vi "Set_Pulse_Single_Channel.vi"(0 "VISA arduino in":refnum<visa-resource-name>, 1 "chanel":u8=2 min=2 max=13 step=1, 2 "Times":dbl[](array[numeric]), 3 "error in":errorcluster, 4 "Check times?":bool) -> (5 "VISA arduino out":refnum<visa-resource-name>, 6 "error out":errorcluster)   [LabVIEW 2021]
uses:
  Delay_Global.vi
  <vilib>/Utility/error.llb/Error Cluster From Error Code.vi
  <vilib>/ErrorRing/Error Ring.xnode
panel:
  out "delay":u32
  # "Private"
  # "Public"
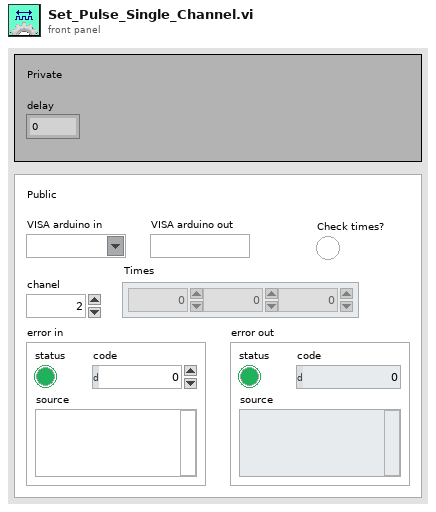
[diagram p1: front panel]
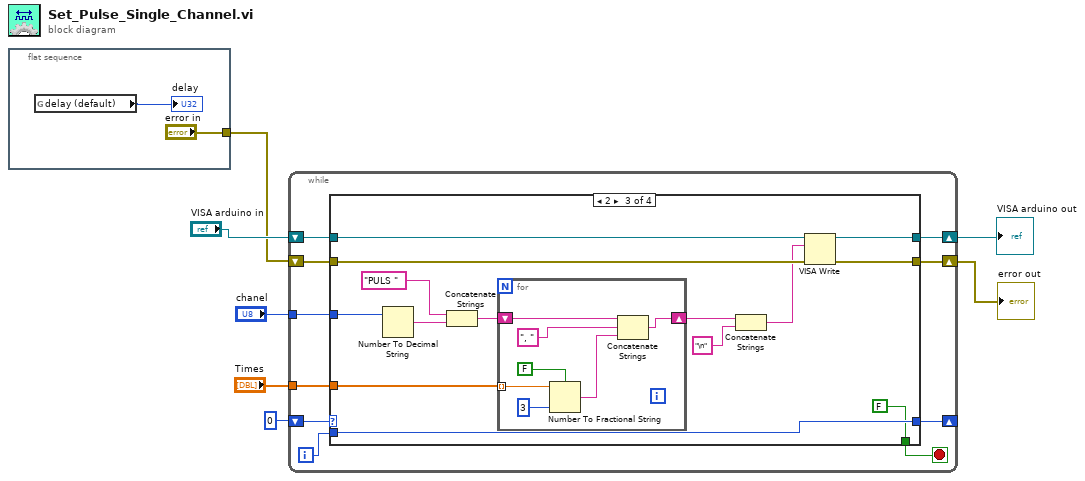
[diagram p0: block diagram]
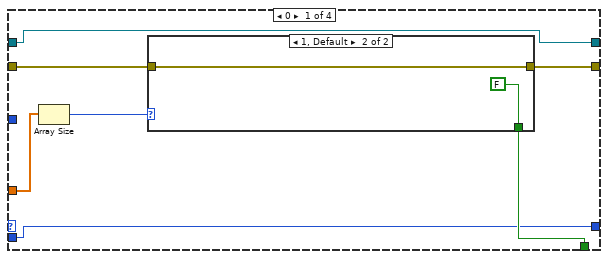
[diagram p2: hidden frame]
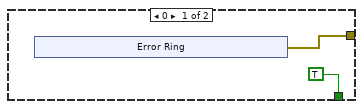
[diagram p3: hidden frame]
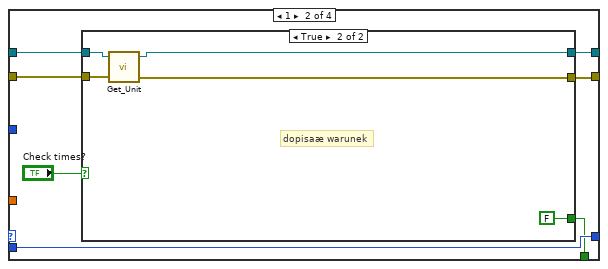
[diagram p4: hidden frame]
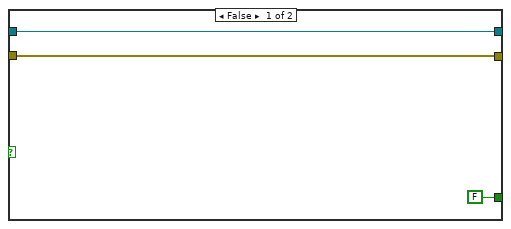
[diagram p5: hidden frame]
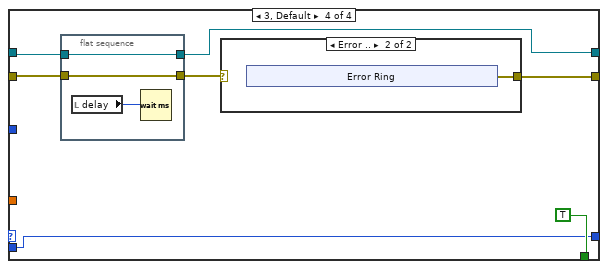
[diagram p6: hidden frame]
diagram:
  n1 = flat-sequence {
    tunnel: ["error in"] -> w1
    frame #0 {
      n2 = global read "Delay_Global.vi" "delay (default)"() -> (→"delay":u32)
    }
  }
  n3 = while {
    shift-right: [w11] -> _
    shift-left: 0 -> [w19]
    tunnel: "Times" -> [w17]
    shift-right: [w12] -> w3
    shift-left: "VISA arduino in" -> [w15]
    shift-right: [w14] -> w2
    shift-left: w1 -> [w16]
    tunnel: "chanel" -> [w10]
    i -> [w18]
    stop <- w13 stop-if-true
    n4 = case shown="2" w19 {
      tunnel: w18 -> [w20 w37 w53 w77]
      tunnel: w17 -> [w26 _ w59 _]
      tunnel: w16 -> [w24 w40 w54 w74]
      tunnel: w15 -> [w21 w41 w55 w72]
      tunnel: [w23 w38 w57 w76] -> w14
      tunnel: [w22 w36 FALSE TRUE] -> w13
      tunnel: [w21 w39 w56 w73] -> w12
      tunnel: [w20 w37 w53 w77] -> w11
      tunnel: w10 -> [_ _ w58 _]
      frame 0 {
        n5 = Array Size(array=w26) -> (size(s)=w25:i32)
        n6 = case shown="1, Default" w25 {
          tunnel: w24 -> [_ w35]
          tunnel: [w28 w35] -> w23
          tunnel: [TRUE FALSE] -> w22
          frame 0 {
            n7 = xnode "Error Ring"() -> ("error out"=w28:errorcluster)
          }
          frame 1, Default {
          }
        }
      }
      frame 1 {
        n8 = case shown="True" "Check times?" {
          tunnel: w41 -> [w45 w50]
          tunnel: w40 -> [w44 w49]
          tunnel: [w45 w48] -> w39
          tunnel: [w44 w47] -> w38
          tunnel: [FALSE FALSE] -> w36
          frame False {
          }
          frame True {
            # "dopisaæ warunek"
            n9 = call "Get_Unit.vi"("error in"=w49, "VISA arduino in"=w50) -> ("error out"=w47:errorcluster, "VISA arduino out"=w48:refnum<visa-resource-name>)  [unwired: 1 in, 1 out]
          }
        }
      }
      frame 2 {
        n10 = Number To Decimal String(number=w58) -> (decimal integer string=w64:string)  [unwired: 1 in]
        n11 = Concatenate Strings("PULS " ("string"), w64) -> (w62:string)
        n12 = for {
          tunnel: w59 -> [w69] mode=indexing
          shift-right: [w71] -> w61
          shift-left: w62 -> [w70]
          n13 = Number To Fractional String(use system decimal point (T)=FALSE, number=w69, precision (6)=i16 3) -> (F-format string=w66:string)  [unwired: 1 in]
          n14 = Concatenate Strings(w70, ", " ("string"), w66) -> (w71:string)
        }
        n15 = Concatenate Strings(w61, "\n" ("string")) -> (w51:string)
        n16 = VISA Write(VISA resource name=w55, write buffer=w51, error in (no error)=w54) -> (VISA resource name out=w56:refnum<visa-resource-name>, error out=w57:errorcluster)  [unwired: 1 out]
      }
      frame 3, Default {
        n17 = flat-sequence {
          tunnel: [w80] -> w75
          tunnel: w74 -> [w80]
          tunnel: [w79] -> w73
          tunnel: w72 -> [w79]
          frame #0 {
            n18 = local read "delay"() -> (w81:u32)
            n19 = Wait (ms)(milliseconds to wait=w81) -> ()  [unwired: 1 out]
          }
        }
        n20 = case shown="Error .." w75 {
          selector: w75 -> [w82 _]
          tunnel: [w82 w83] -> w76
          frame No Error {
          }
          frame Error {
            n21 = xnode "Error Ring"() -> ("error out"=w83:errorcluster)
          }
        }
      }
    }
  }
  "error out" <- w2
  "VISA arduino out" <- w3
